vi "findObj.vi"(10 "inputObjName":string, 11 "inputObjArray":T1[](array[typedef])) -> (1 "index":i32, 2 "found?":bool, 3 "outputObj":T1)   [LabVIEW 2015]
uses:
  processedObjectInfo.ctl
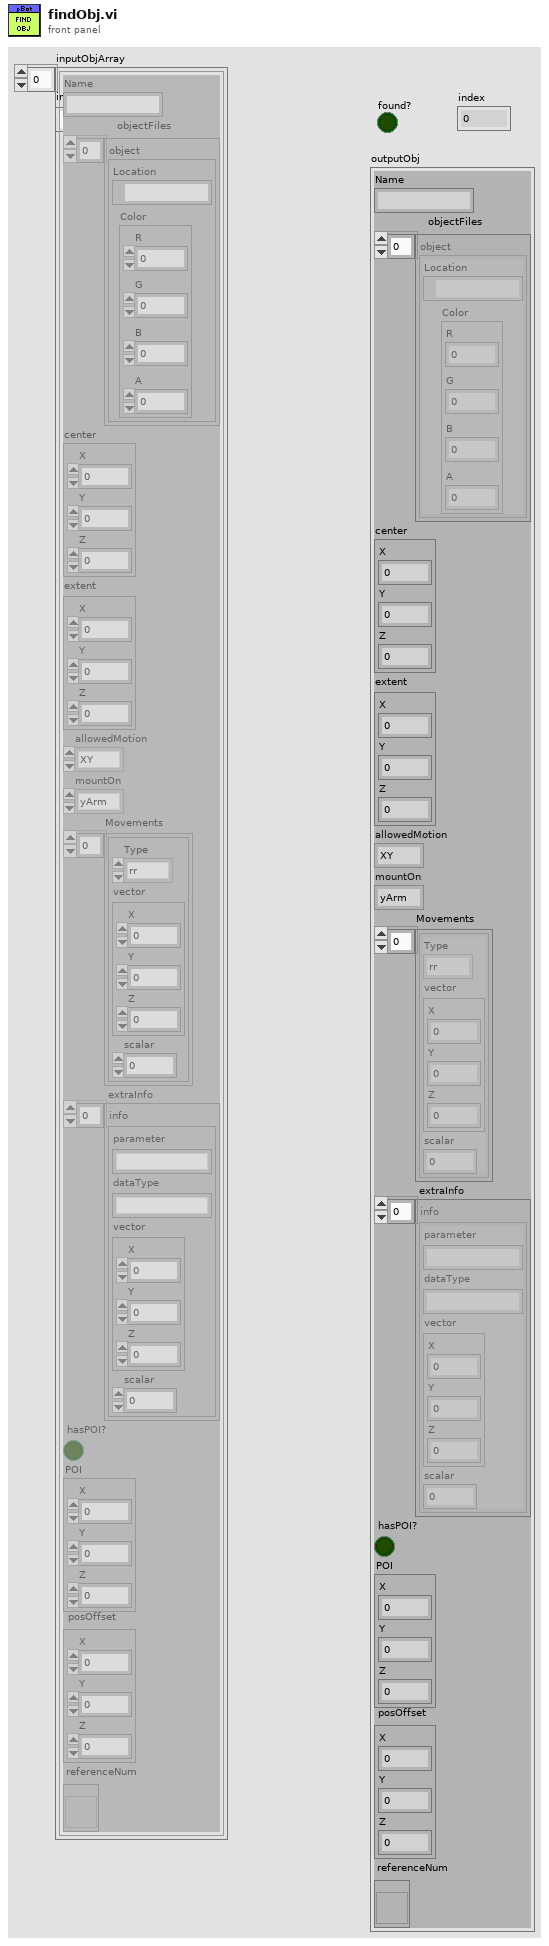
[diagram p1: front panel]
types:
  T1 = typedef "processedObjectInfo.ctl" = cluster{"Name":string, "objectFiles":cluster{"Location":path, "Color":cluster{"R":dbl, "G":dbl, "B":dbl, "A":dbl}}[], "center":cluster{"X":dbl, "Y":dbl, "Z":dbl}, "extent":cluster{"X":dbl, "Y":dbl, "Z":dbl}, "allowedMotion":enum16{"XY", "Z"}, "mountOn":enum16{"yArm", "breadBoard"}, "Movements":cluster{"Type":enum16{"rr", "ra", "tr", "ta"}, "vector":cluster{"X":dbl, "Y":dbl, "Z":dbl}, "scalar":dbl}[], "extraInfo":cluster{"parameter":string, "dataType":string, "vector":cluster{"X":dbl, "Y":dbl, "Z":dbl}, "scalar":dbl}[], "hasPOI?":bool, "POI":cluster{"X":dbl, "Y":dbl, "Z":dbl}, "posOffset":cluster{"X":dbl, "Y":dbl, "Z":dbl}, "referenceNum":refnum<vi>}
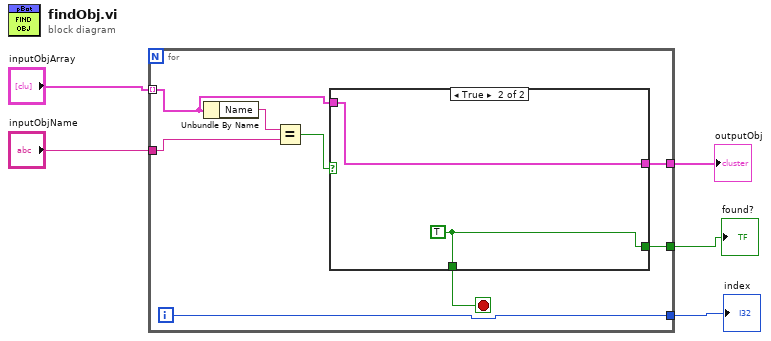
[diagram p0: block diagram]
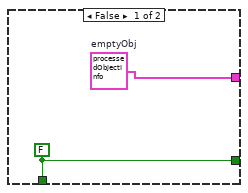
[diagram p2: hidden frame]
diagram:
  n1 = for {
    tunnel: "inputObjArray" -> [w9] mode=indexing
    tunnel: "inputObjName" -> [w13]
    tunnel: [w10] -> w1
    tunnel: [w7] -> w3
    tunnel: [w6] -> w2
    i -> [w6]
    stop <- w8 stop-if-true
    n2 = Unbundle By Name(w9) -> ("Name"=w12:string)
    n3 = Equal?(x=w12, y=w13) -> (x = y?=w11:bool)
    n4 = case shown="True" w11 {
      tunnel: [w14 w16] -> w10
      tunnel: w9 -> [_ w16]
      tunnel: [w15 w17] -> w8
      tunnel: [w15 w17] -> w7
      frame False {
        w14 = T1 {"Name"="", "objectFiles"=[], "center"={"X"=0.0, "Y"=0.0, "Z"=0.0}, "extent"={"X"=0.0, "Y"=0.0, "Z"=0.0}, "allowedMotion"=enum."XY", "mountOn"=enum."yArm", "Movements"=[], "extraInfo"=[], "hasPOI?"=FALSE, "POI"={"X"=0.0, "Y"=0.0, "Z"=0.0}, "posOffset"={"X"=0.0, "Y"=0.0, "Z"=0.0}, "referenceNum"=refnum}  # emptyObj
        w15 = FALSE
      }
      frame True {
        w17 = TRUE
      }
    }
  }
  "outputObj" <- w1
  "found?" <- w3
  "index" <- w2
